vi "Shooter.vi"() -> ()   [LabVIEW 2013]
uses:
  <vilib>/Rock Robotics/SystemInterfaces/DIO/FPGA_DIOPWMChannel.ctl
  <vilib>/Rock Robotics/WPI/MotorControl/WPI_MotorControlOpen Talon.vi
panel:
  in  "Return":bool
  in  "Fire":bool
  in  "State Control":enum16{"Open", "Run", "End"}(ring)
  in  "Encoder":dbl
  in  "4 Feet":bool
  in  "2 Feet":bool
  in  "4 Feet 2":dbl=200.0 format="%#_13g"
  in  "2 Feet 2":dbl=100.0 format="%#_13g"
  in  "Manual Shoot":bool
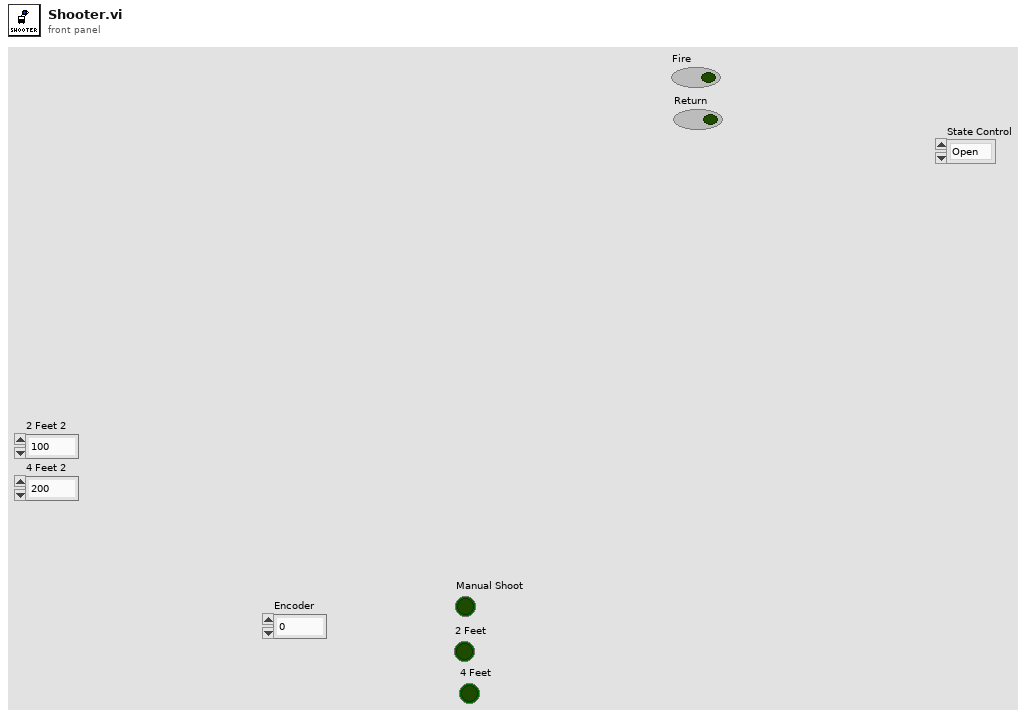
[diagram p1: front panel]
types:
  T1 = typedef "FPGA_DIOPWMChannel.ctl" = enum8{"PWM 1", "PWM 2", "PWM 3", "PWM 4", "PWM 5", "PWM 6", "PWM 7", "PWM 8", "PWM 9", "PWM 10", "Invalid"}
  T2 = typedef "WPI_MotorControlDeviceRef.ctl" = cluster{"DeviceStatus":errorcluster, "Type":enum16{"PWM", "CAN"}, "PWM":cluster{"Digital Module":T3, "PWM Channel":T1, "DeadBand":T4}, "CAN":cluster{"Device Number":u8, "Control Mode":T5, "Semaphore":T6, "Max Vout":dbl}, "Invert":bool, "TransformRef":T7, "InvTransformRef":T7}
  T3 = typedef "FPGA_TypedefDigitalModule.ctl" = enum16{"Digital Module 1", "Digital Module 2"}
  T4 = typedef "WPI_PWMDeadband.ctl" = cluster{"Name":string, "maxPositivePwm":i32, "minPositivePwm":i32, "centerPwm":i32, "maxNegativePwm":i32, "minNegativePwm":i32, "angularRange":u16}
  T5 = typedef "WPI_CANJaguar_ControlMode.ctl" = enum8{"Percent VBus", "Current", "Speed", "Position", "Voltage"}
  T6 = typedef "Semaphore RefNum" = refnum<k1>
  T7 = typedef "WPI_PWMTransform_ConPane.ctl" = refnum<vi>
  T8 = enum16{"No Shoot", "Manual Shoot", "2 Feet", "4 Feet"}
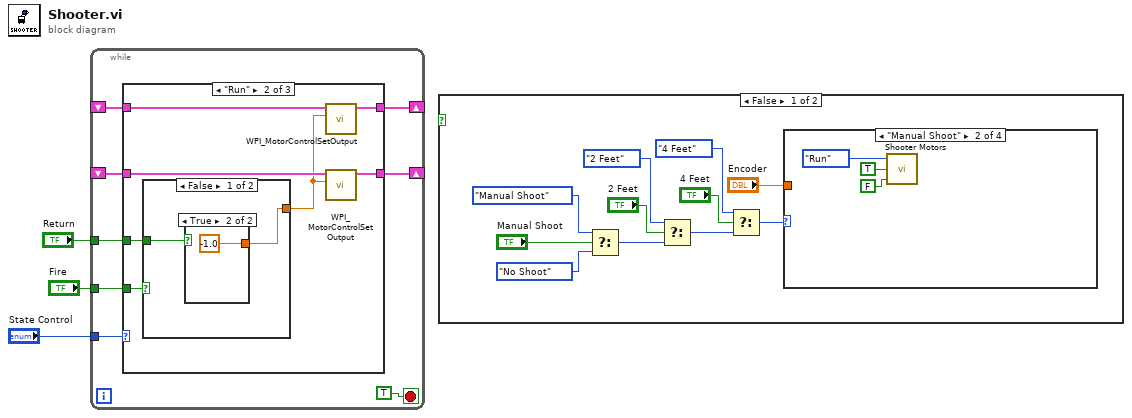
[diagram p0: block diagram]
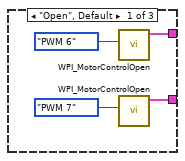
[diagram p2: hidden frame]
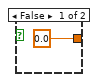
[diagram p3: hidden frame]
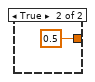
[diagram p4: hidden frame]
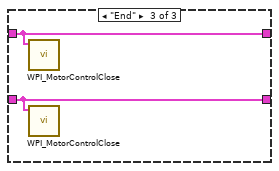
[diagram p5: hidden frame]
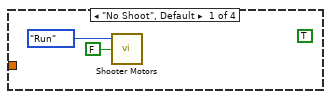
[diagram p6: hidden frame]
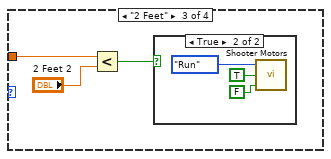
[diagram p7: hidden frame]
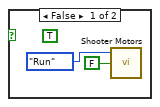
[diagram p8: hidden frame]
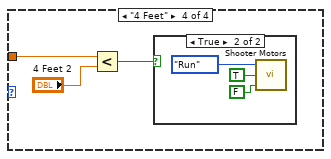
[diagram p9: hidden frame]
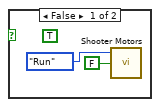
[diagram p10: hidden frame]
diagram:
  n1 = while {
    shift-right: [w11] -> _
    shift-left: _ -> [w10]
    tunnel: "State Control" -> [w9]
    shift-right: [w7] -> _
    shift-left: _ -> [w6]
    tunnel: "Fire" -> [w5]
    tunnel: "Return" -> [w4]
    stop <- TRUE stop-if-true
    n2 = case shown="\"Run\"" w9 {
      tunnel: [w13 w19 w29] -> w11
      tunnel: w10 -> [_ w21 w29]
      tunnel: [w12 w18 w28] -> w7
      tunnel: w6 -> [_ w22 w28]
      tunnel: w5 -> [_ w17 _]
      tunnel: w4 -> [_ w16 _]
      frame "Open", Default {
        n3 = call-poly <vilib>:"WPI_MotorControlOpen.vi"("PWM Channel"=FPGA_DIOPWMChannel."PWM 6" ("PWMChannel")) -> ("MotorControlDeviceRef"=w13:T2)  [unwired: 9 in, 1 out]
        n4 = call-poly <vilib>:"WPI_MotorControlOpen.vi"("PWM Channel"=FPGA_DIOPWMChannel."PWM 7" ("PWMChannel")) -> ("MotorControlDeviceRef"=w12:T2)  [unwired: 9 in, 1 out]
      }
      frame "Run" {
        n5 = case shown="False" w17 {
          tunnel: [w23 0.5 ("Output")] -> w20
          tunnel: w16 -> [w24 _]
          frame False {
            n6 = case shown="True" w24 {
              tunnel: [0.0 -1.0] -> w23
              frame False {
              }
              frame True {
              }
            }
          }
          frame True {
          }
        }
        n7 = call <vilib>:"WPI_MotorControlSetOutput.vi"("Output"=w20, "MotorControlDevRef"=w21) -> ("MotorControlDevRef"=w19:T2)  [unwired: 7 in, 2 out]
        n8 = call <vilib>:"WPI_MotorControlSetOutput.vi"("Output"=w20, "MotorControlDevRef"=w22) -> ("MotorControlDevRef"=w18:T2)  [unwired: 7 in, 2 out]
      }
      frame "End" {
        n9 = call <vilib>:"WPI_MotorControlClose.vi"("MotorControlDevRef"=w29) -> ()  [unwired: 10 in, 1 out]
        n10 = call <vilib>:"WPI_MotorControlClose.vi"("MotorControlDevRef"=w28) -> ()  [unwired: 10 in, 1 out]
      }
    }
  }
  n11 = case shown="\"New\"" {
    selector: _ -> [_ _]
    frame False {
      n12 = Select(t=T8."Manual Shoot" ("Shoot 2"), s="Manual Shoot", f=T8."No Shoot" ("Shoot 2")) -> (s? t:f=w34:T8)
      n13 = Select(t=T8."2 Feet" ("Shoot 2"), s="2 Feet", f=w34) -> (s? t:f=w37:T8)
      n14 = Select(t=T8."4 Feet" ("Shoot 2"), s="4 Feet", f=w37) -> (s? t:f=w39:T8)
      n15 = case shown="\"Manual Shoot\"" w39 {
        tunnel: "Encoder" -> [_ _ w47 w54]
        frame "No Shoot", Default {
          (unwired) TRUE ("Return")
          n16 = call "Shooter Motors.vi"("Fire"=FALSE, "State Control"=enum16{"Open", "Run", "End"}."Run") -> ()  [unwired: 1 in]
        }
        frame "Manual Shoot" {
          n17 = call "Shooter Motors.vi"("Return"=FALSE, "Fire"=TRUE, "State Control"=enum16{"Open", "Run", "End"}."Run") -> ()
        }
        frame "2 Feet" {
          n18 = Less?(x=w47, y="2 Feet 2") -> (x < y?=w46:bool)
          n19 = case shown="True" w46 {
            frame False {
              (unwired) TRUE ("Return")
              n20 = call "Shooter Motors.vi"("Fire"=FALSE, "State Control"=enum16{"Open", "Run", "End"}."Run") -> ()  [unwired: 1 in]
            }
            frame True {
              n21 = call "Shooter Motors.vi"("Return"=FALSE, "Fire"=TRUE, "State Control"=enum16{"Open", "Run", "End"}."Run") -> ()
            }
          }
        }
        frame "4 Feet" {
          n22 = Less?(x=w54, y="4 Feet 2") -> (x < y?=w55:bool)
          n23 = case shown="True" w55 {
            frame False {
              (unwired) TRUE ("Return")
              n24 = call "Shooter Motors.vi"("Fire"=FALSE, "State Control"=enum16{"Open", "Run", "End"}."Run") -> ()  [unwired: 1 in]
            }
            frame True {
              n25 = call "Shooter Motors.vi"("Return"=FALSE, "Fire"=TRUE, "State Control"=enum16{"Open", "Run", "End"}."Run") -> ()
            }
          }
        }
      }
    }
    frame True {
    }
  }
